vi "Delete Panel Data.vi"(8 "Error In":errorcluster, 10 "Field":string, 11 "Panel Helper in":refnum<class "Panel Helper.lvclass">) -> (0 "Error Out":errorcluster, 2 "Found?":bool)   [LabVIEW 2020, in "Panel.lvlib" / "Panel Helper.lvclass"]
doc: "Deletes a field from the Panel Data\n\n<B>Panel Helper In:</B> Panel Helper object to write panel data\n<B>Field:</B> Data field associated with the panel data.\n<B>Error In:</B> Describes error conditions that occur before this node runs.\n\n<B>Found?:</B> Indicates if the Panel Data was found.\n<B>Error Out:</B> Contains error information.\n----\nPlease see the following web address for additional documentation and tutorial information:\nhttp://www.mooregoodideas.com/mgi-panel-manager/\n\nAuthor: Derek Trepanier\n\nCopyright (c) 2018, Moore Good Ideas, Inc.\n\nAll rights reserved.\n\nRedistribution and use in source and binary forms, with or without modification, are permitted provided that the following conditions are met:\n\n * Redistributions of source code must retain the above copyright notice, this list of conditions and the following disclaimer.\n * Redistributions in binary form must reproduce the above copyright notice, this list of conditions and the following disclaimer in the documentation and/or other materials provided with the distribution.\n * Neither the name of Moore Good Ideas, Inc. nor the names of its contributors may be used to endorse or promote products derived from this software without specific prior written permission.\n\nTHIS SOFTWARE IS PROVIDED BY THE COPYRIGHT HOLDERS AND CONTRIBUTORS \"AS IS\" AND ANY EXPRESS OR IMPLIED WARRANTIES, INCLUDING, BUT NOT LIMITED TO, THE IMPLIED WARRANTIES OF MERCHANTABILITY AND FITNESS FOR A PARTICULAR PURPOSE ARE DISCLAIMED. IN NO EVENT SHALL THE COPYRIGHT OWNER OR CONTRIBUTORS BE LIABLE FOR ANY DIRECT, INDIRECT, INCIDENTAL, SPECIAL, EXEMPLARY, OR CONSEQUENTIAL DAMAGES (INCLUDING, BUT NOT LIMITED TO, PROCUREMENT OF SUBSTITUTE GOODS OR SERVICES; LOSS OF USE, DATA, OR PROFITS; OR BUSINESS INTERRUPTION) HOWEVER CAUSED AND ON ANY THEORY OF LIABILITY, WHETHER IN CONTRACT, STRICT LIABILITY, OR TORT (INCLUDING NEGLIGENCE OR OTHERWISE) ARISING IN ANY WAY OUT OF THE USE OF THIS SOFTWARE, EVEN IF ADVISED OF THE POSSIBILITY OF SUCH DAMAGE."
uses:
  <vilib>/MGI/Panel Manager/Panel/Panel Helper/Panel Helper.lvclass
  <vilib>/MGI/Panel Manager/Panel/Panel Helper/Panel Helper.lvclass/Panel Helper.ctl
  <vilib>/MGI/Panel Manager/Panel/Panel Updater/Panel Updater.lvclass
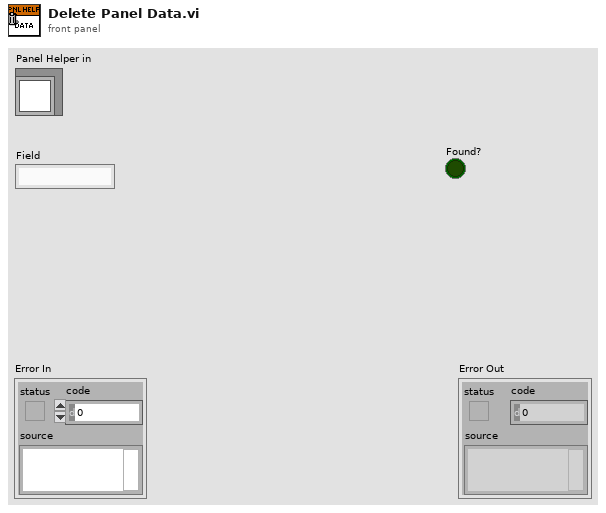
[diagram p1: front panel]
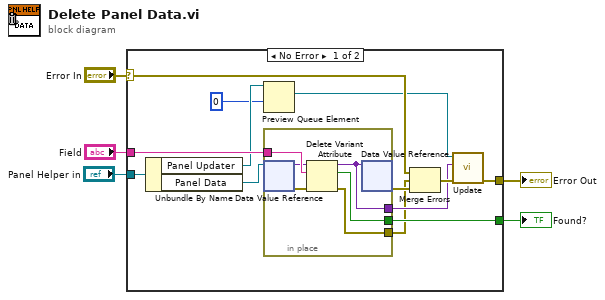
[diagram p0: block diagram]
diagram:
  n1 = case shown="No Error" "Error In" {
    selector: "Error In" -> [w18 w25]
    tunnel: [w14 w25] -> w2
    tunnel: "Panel Helper in" -> [w17 _]
    tunnel: [w15 _] -> w1
    tunnel: "Field" -> [w13 _]
    frame No Error {
      n2 = Unbundle By Name(w17) -> ("Panel Updater"=w8:refnum<queue>, "Panel Data"=w16:refnum<data-value>)
      n3 = Preview Queue Element(queue=w8, timeout in ms (-1)=0) -> (element=w7:refnum<class "Panel Updater.lvclass">)  [unwired: 1 in, 3 out]
      n4 = in-place {
        in-place-border: w13 -> [w20]
        in-place-border: [w24] -> w15
        in-place-border: [w22] -> w9
        in-place-border: [w21] -> w10
        n5 = in-place-dvr #1(w16) -> (w19:variant, w23:errorcluster)
        n6 = Delete Variant Attribute(4:w23, 6:w20, 7:w19) -> (0:w22:errorcluster, 2:w24:bool, 3:w21:variant)
        n7 = in-place-dvr #1(w21) -> (w11:errorcluster)  [unwired: 1 out]
      }
      n8 = Merge Errors(w18, w9, w11) -> (w12:errorcluster)
      n9 = call-dynamic "Update.vi"("error in (no error)"=w12, "Panel Data"=w10, "Panel Updater in"=w7) -> ("error out"=w14:errorcluster)  [unwired: 8 in]
    }
    frame Error {
    }
  }
  "Error Out" <- w2
  "Found?" <- w1
